vi "二极管.vi"() -> ()   [LabVIEW 2021]
panel:
  out "XY Graph":cluster{"Y":dbl[], "Y":dbl[]}[](graph)
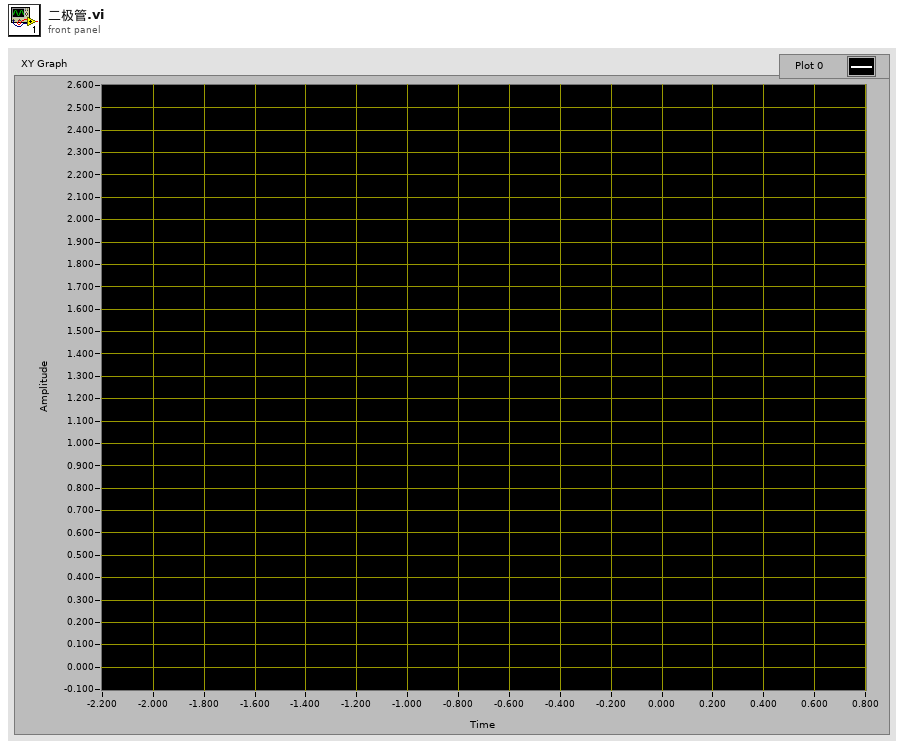
[diagram p1: front panel]
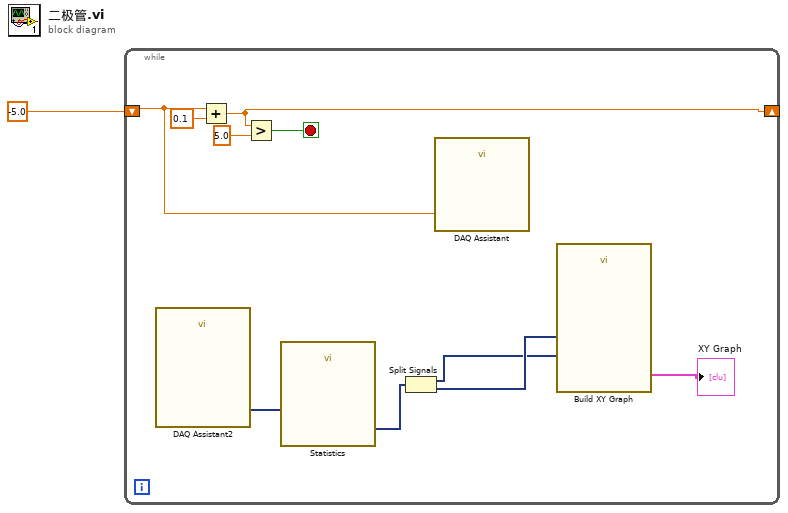
[diagram p0: block diagram]
diagram:
  n1 = while {
    shift-right: [w7] -> _
    shift-left: -5.0 -> [w5]
    stop <- w9 stop-if-true
    n2 = call "DAQ Assistant2"() -> ("data"=w3:dynamicdata)  [unwired: 17 in, 2 out]
    n3 = Add(x=w5, y=0.1) -> (x+y=w7:dbl)
    n4 = Greater?(x=w7, y=5.0) -> (0:w9:bool)
    n5 = call "Statistics"("Signals"=w3) -> ("Arithmetic Mean"=w4:dynamicdata)  [unwired: 25 in, 1 out]
    n6 = Split Signals(w4) -> (w2:dynamicdata, w6:dynamicdata)  [unwired: 2 in]
    n7 = call "DAQ Assistant"("data"=w5) -> ()  [unwired: 17 in, 2 out]
    n8 = call "Build XY Graph"("Y Input"=w2, "X Input"=w6) -> ("XY Graph"=→"XY Graph":cluster{"X":dbl[], "Y":dbl[]}[])  [unwired: 8 in, 1 out]
  }
